vi "GV detector trigger.vi"() -> ()   [LabVIEW 2017]
panel:
  in  "Detector trigger":bool
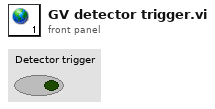
[diagram p1: front panel]
diagram:
